vi "AMZ_S3_ERR_Check if Error Occured.vi"(8 "error in (no error)":errorcluster, 11 "Response header":string) -> (0 "error out":errorcluster, 2 "500 Error?":bool, 3 "Error Occured?":bool)   [LabVIEW 2015, in "LV Interface for Amazon S3.lvlib"]
doc: "Check the response header to see if there was an error.\nIf an error is found, the AWS_S3_Get_Call_Result.vi may get the details from the response body."
uses:
  LV Interface for Amazon S3.lvlib
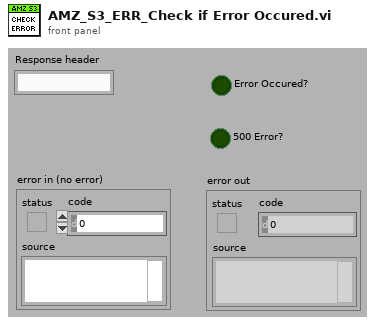
[diagram p1: front panel]
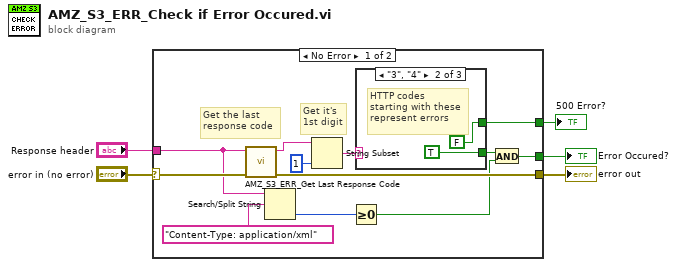
[diagram p0: block diagram]
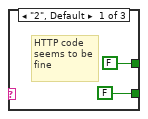
[diagram p2: hidden frame]
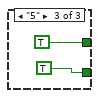
[diagram p3: hidden frame]
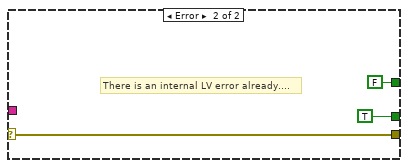
[diagram p4: hidden frame]
diagram:
  n1 = case shown="No Error" "error in (no error)" {
    selector: "error in (no error)" -> [w13 w26]
    tunnel: [w12 w26] -> w3
    tunnel: "Response header" -> [w8 _]
    tunnel: [w14 TRUE] -> w2
    tunnel: [w6 FALSE] -> w1
    frame No Error {
      # "Get it's\n1st digit"
      # "Get the last\nresponse code"
      n2 = call "AMZ_S3_ERR_Get Last Response Code.vi"("error in (no error)"=w13, "Response header"=w8) -> ("error out"=w12:errorcluster, "Response code (last)"=w11:string)  [unwired: 8 in]
      n3 = Search/Split String(string=w8, search string/char (-)="Content-Type: application/xml") -> (offset of match=w16:i32)  [unwired: 1 in, 2 out]
      n4 = String Subset(string=w11, length (rest)=1 ("length (rest)")) -> (substring=w10:string)  [unwired: 1 in]
      n5 = Greater Or Equal To 0?(x=w16) -> (x >= 0?=w7:bool)
      n6 = case shown="\"3\", \"4\"" w10 {
        tunnel: [FALSE TRUE TRUE] -> w15
        tunnel: [FALSE FALSE TRUE] -> w6
        frame "2", Default {
          # "HTTP code\nseems to be\nfine"
        }
        frame "3", "4" {
          # "HTTP codes\nstarting with these\nrepresent errors"
        }
        frame "5" {
        }
      }
      n7 = And(x=w15, y=w7) -> (x .and. y?=w14:bool)
    }
    frame Error {
      # "There is an internal LV error already...."
    }
  }
  "Error Occured?" <- w2
  "error out" <- w3
  "500 Error?" <- w1
